vi "RGB To YCbCr (SubVI).vi"(11 "Image Out":T1 {"Dialogs" format="%.0b"}) -> (1 "Cb":dbl[][](array[numeric]), 2 "Cr":dbl[][](array[numeric]), 3 "y":dbl[][](array[numeric]))   [LabVIEW 2012]
uses:
  <userlib>/ImageProcessing/QTLIB_2595_LV86/QT_Image.ctl
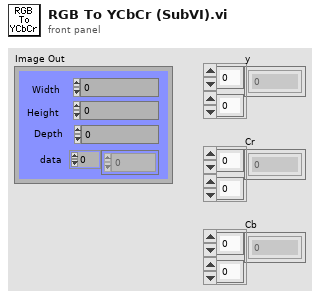
[diagram p1: front panel]
types:
  T1 = typedef "QT_Image.ctl" = cluster{"Width":i32, "Height":i32, "Depth":i32, "data":u8[], "Compressed data":u8[], "Color table":u32[], "Duration":i32, "Options":i32, "Timestamp":i32, "ID":i32, "Reserved":i32, "Dialogs":u32}
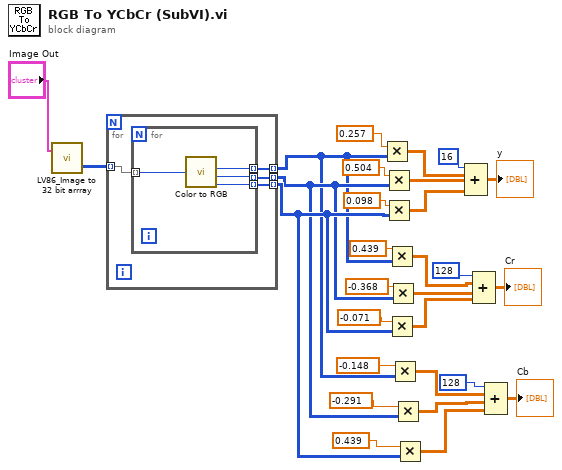
[diagram p0: block diagram]
diagram:
  n1 = call <userlib>:"LV86_Image to 32 bit arrray.vi"("Image In"="Image Out") -> ("Intensity Graph"=w2:u32[][])  [unwired: 1 in, 1 out]
  n2 = for {
    tunnel: w2 -> [w33] mode=indexing
    tunnel: [w32] -> w3 mode=indexing
    tunnel: [w31] -> w4 mode=indexing
    tunnel: [w30] -> w5 mode=indexing
    n3 = for {
      tunnel: w33 -> [w37] mode=indexing
      tunnel: [w36] -> w32 mode=indexing
      tunnel: [w35] -> w31 mode=indexing
      tunnel: [w34] -> w30 mode=indexing
      n4 = call <vilib>:"Color to RGB.vi"("Color"=w37) -> ("R"=w36:u8, "G"=w35:u8, "B"=w34:u8)  [unwired: 1 out]
    }
  }
  n5 = Multiply(x=0.257, y=w3) -> (x*y=w9:dbl[][])
  n6 = Multiply(x=0.504, y=w4) -> (x*y=w10:dbl[][])
  n7 = Multiply(x=0.098, y=w5) -> (x*y=w11:dbl[][])
  n8 = Multiply(x=0.439, y=w3) -> (x*y=w20:dbl[][])
  n9 = Multiply(x=-0.071, y=w5) -> (x*y=w22:dbl[][])
  n10 = Multiply(x=-0.368, y=w4) -> (x*y=w21:dbl[][])
  n11 = Multiply(x=-0.148, y=w3) -> (x*y=w25:dbl[][])
  n12 = Multiply(x=-0.291, y=w4) -> (x*y=w26:dbl[][])
  n13 = Multiply(x=0.439, y=w5) -> (x*y=w27:dbl[][])
  n14 = Compound Arithmetic op=ADD(16, w9, w10, w11) -> (→"y":dbl[][])
  n15 = Compound Arithmetic op=ADD(128, w20, w21, w22) -> (→"Cr":dbl[][])
  n16 = Compound Arithmetic op=ADD(128, w25, w26, w27) -> (→"Cb":dbl[][])
